vi "dataAcq_get_spectrum.vi"(0 "reference":refnum<class "OSA.lvclass">, 5 "error in (no error)":errorcluster, 9 "x data create":bool) -> (14 "duplicate reference":refnum<class "OSA.lvclass">, 19 "error out":errorcluster)   [LabVIEW 2010, in "OSA.lvclass"]
doc: "Reads data from spectrometer and updates labview buffer spectrum Y array, X is either equidistant, (x min and max), or contains a full X-array. See buffer_get.vi for labview buffer data access.\n\nX: periods/cm\nY: mW absolute pwr, (pwr/resolution)"
uses:
  OSA.lvclass
  typeDef/xVal_option.ctl
  OSA20X_misc.lvlib
  FTSLib.dll
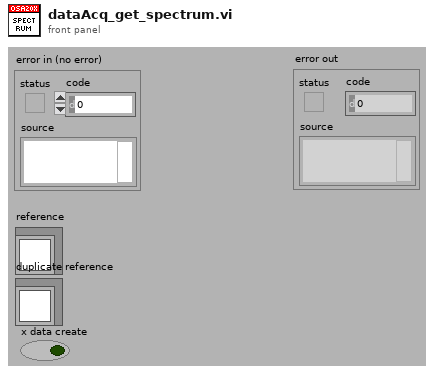
[diagram p1: front panel]
types:
  T1 = enum16{"get", "init", "set interferogram", "set spectrum", "cleanUp"}
  T2 = typedef "OSA.lvclass/ObjectAttributes.ctl" = cluster{"Stop":bool, "dataType":T3, "spectrometerIdx":u16, "buffer size interferogram":i32, "interferogram":cluster{"new":bool, "plot_x_ min":sgl, "plot_x_max":sgl, "plot_y_min":sgl, "plot_y_max":sgl, "Graph Intrfrgrm":T4, "timeStamp":u32, "signal (%)":dbl, "traces":cluster{"idx":u32, "broadBand":bool, "monoChromatic":bool, "peakToPeakSignal":dbl, "peakToPeakPos":dbl}[], "traces idx last":i32}, "spectrum":cluster{"new":bool, "plot_x_min":sgl, "plot_x_max":sgl, "plot_unit_x":T5, "plot_unit_y":T6, "plot_y_min":sgl, "plot_y_max":sgl, "Graph Spectrum":T4, "timeStamp":u32, "X_VAL_OPTIONS":enum16{"MIN_MAX", "ARRAY"}, "traces":cluster{"idx":u32}[], "traces idx last":i32}, "Thorlabs_OSA_64.lvclass:queue_action.ctlqueue ref":refnum<queue>, "action":T7, "plot zoom step":dbl, "buffer semaphore":T8, "acq stopped":bool, "dataType active":T3, "temperature (degr C)":sgl, "pressure (hPa)":sgl, "rel humidity (%)":sgl, "settings":cluster{"resolution":T9, "sensitivity":T10, "Average":bool, "average nr":u32, "apodisation":T11, "acq delay (ms)":u32, "airMesure":T12, "wmtr on":bool, "intfgrm_smooth_width":u16, "intfgrm_smooth_nrOfPasses":u16, "intfgrm_smooth":T13, "phaseCorrection":T14, "zeroFill":u8, "spectr_smooth":T13, "spectr_smooth_width":u16, "spectr_smooth_nrOfPasses":u16, "resolution (/cm)":sgl, "REF wavelength, (nm)":dbl, "gain_idx":u16, "gainAuto":bool, "gain_relative":dbl, "PD sensitivity mode":T15, "PD senseMode implemented":bool, "SensorTemperature implemented":bool, "SensorPressure implemented":bool, "SensorHumidity implemented":bool}, "peaks position":sgl[], "peaks width":sgl[], "peaks height":sgl[], "peaks max nr":u32, "peaks latest nr":i32, "peaks new":bool, "power":dbl, "power new":bool, "path":string, "wavelength (WNr)":dbl, "wavelength new":bool, "buffer size spectrum":i32, "status":string, "VI reference":refnum<vi>, "funcPointer":u64, "libraryPointer":u64, "singleAcquisition":bool, "coherenceLength (cm)":dbl, "coherenceLength new":bool, "spectrometer model":string, "spectrometer serial nr":string, "peaks thld left":sgl[], "peaks thld right":sgl[], "coherenceLength error (cm)":dbl, "ADC bits":u16, "peaks position centroid":sgl[], "peaks height centroid":sgl[], "OSA series":T16, "channel index":u16, "channel index stiched":u16, "spectrum channel type":T17}
  T3 = typedef "OSA.lvclass/acq_dataType.ctl" = enum16{"none", "interferogram", "spectrum"}
  T4 = typedef "OSA.lvclass/graph_intensity.ctl" = refnum<vi>
  T5 = typedef "OSA.lvclass/spectrum_x_unit.ctl" = enum16{"wavenr/cm", "THz", "eV", "nm_air", "nm_vac"}
  T6 = typedef "OSA.lvclass/y_unit.ctl" = enum16{"ADC counts", "dBm pwr absolute", "dBm pwr density", "mW pwr absolute", "mW pwr density"}
  T7 = typedef "OSA.lvclass/queue_action.ctl" = enum16{"none", "stop", "GUI_plotInterferogram", "GUI_plotSpectrum", "GUI_plotInterferogramRescale", "GUI_plotSpectrumRescale", "GUI_plotInterferogramReset", "GUI_plotSpectrumReset", "GUI_plotInterferogramAutoScaleY", "GUI_plotSpectrumAutoScaleY", "GUI_plotInterferogramZoomOut", "GUI_plotSpectrumZoomOut", "GUI_plotInterferogramPane", "GUI_plotSpectrumPane", "GUI_plotInterferogramZoomMouse", "GUI_plotSpectrumZoomMouse", "ENVIRONMENT temperature", "ENVIRONMENT pressure", "MODE_resolution set", "MODE_resolution get", "MODE_sensitivity set", "MODE_sensitivity get", "MODE_PDTemperature set", "MODE_PDTemperature get", "REBOOT/RESET firmware", "ACQASYNC_acquireSingleSpectrum", "ACQASYNC_continuous start", "ACQASYNC_continuous stop\n", "ACQASYNC_get last interferogram", "ACQASYNC_get last spectrum", "ACQASYNC_get last waveNr", "ACQOPT_interferogram smoothing set", "ACQOPT_interferogram smoothing get", "ACQOPT_spectrum smoothing set", "ACQOPT_spectrum smoothing get", "ACQOPT_apodisation type set", "ACQOPT_apodisation type get", "ACQOPT_phase correction type set", "ACQOPT_phase correction type get", "ACQOPT_acqIntervall_set", "ACQOPT_acqIntervall_get", "ACQOPT_average spectrum set", "ACQOPT_average spectrum get", "ACQOPT_rolling average set", "ACQOPT_rolling average get", "ACQOPT_zero fill factor set", "ACQOPT_zero fill factor get", "ACQOPT_cycle counting set", "ACQOPT_cycle counting get", "ACQOPT_air measure option set", "ACQOPT_air measure option get", "ACQOPT_gainLevel auto get", "ACQOPT_gainLevel auto set", "ACQOPT_gainLevel get", "ACQOPT_gainLevel set", "ACQOPT_getAll", "INSTRUMENT_PROPERTY_range_WaveNr_min", "INSTRUMENT_PROPERTY_range_WaveNr_max", "INSTRUMENT_PROPERTY_reference_wavelength_cm^-1", "INSTRUMENT_PROPERTY_samplesPerRefPeriod", "INSTRUMENT_PROPERTY_resolution_waveNrPercm", "INSTRUMENT_PROPERTY_availableGainLevels", "INSTRUMENT_PROPERTY_status", "CONVERT", "ANALYSE_POWER", "ANALYSE_PEAKS", "ANALYSE_WAVELENGTH", "ANALYSE_SPECTRUM", "ANALYSE_INTERFEROGRAM", "ANALYSE_COHERENCE_LENGTH", "MATH", "MATH_power", "MATH_peaks", "FILE", "miscellaneous"}
  T8 = typedef "Semaphore RefNum" = refnum<k1>
  T9 = typedef "OSA.lvclass/resolution.ctl" = enum16{"low", "high"}
  T10 = typedef "OSA.lvclass/sensitivityMode.ctl" = enum16{"low", "low medium", "high medium", "high"}
  T11 = typedef "OSA.lvclass/apodisation.ctl" = enum16{"NONE", "NORTON_BEER_WEAK", "NORTON_BEER_MEDIUM", "NORTON_BEER_STRONG", "TRIANGULAR", "COSINE", "HANN", "HAMMING", "BLACKMANHARRIS3", "BLACKMANHARRIS4", "GAUSSIAN"}
  T12 = typedef "OSA.lvclass/airMeasure.ctl" = enum16{"TEMPERATURE", "PRESSURE"}
  T13 = typedef "OSA.lvclass/smoothing.ctl" = enum16{"NONE", "BINOMIAL", "SAVITSKY_GOLAY", "FOURIER", "MOVING_AVERAGE", "GAUSSIAN"}
  T14 = typedef "OSA.lvclass/phaseCorrection.ctl" = enum16{"NONE", "MERTZ", "FORMAN", "MERTZ_FILE", "FORMAN_FILE", "FUTURE COMP."}
  T15 = typedef "OSA.lvclass/PDTemperatureMode.ctl" = enum16{"cool: better sensitivity/noise floor", "warm: extended wl range"}
  T16 = typedef "OSA.lvclass/OSA_series.ctl" = enum16{"OSA200", "OSA300", "UNKNOWN"}
  T17 = typedef "OSA.lvclass/channelType_spectrum.ctl" = enum16{"SINGLE CHANNEL", "STICHED"}
  T18 = typedef "OSA.lvclass/xVal_option.ctl" = enum16{"MIN_MAX", "ARRAY"}
  T19 = cluster{"length":u32, "X min":sgl, "X max":sgl, "X_VAL_OPTIONS":T18}
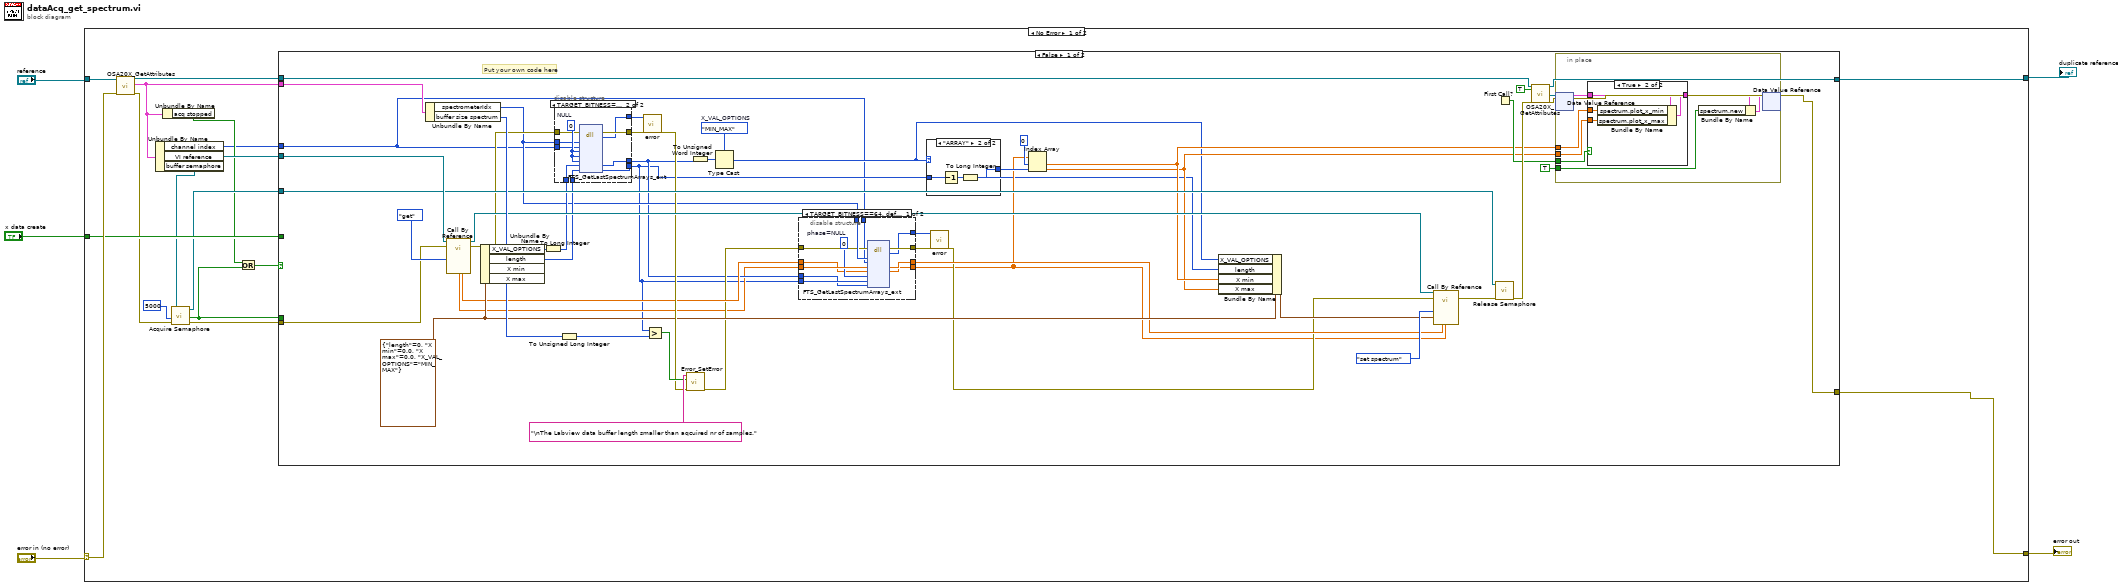
[diagram p0: block diagram]
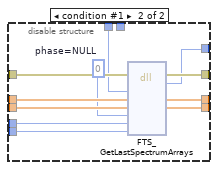
[diagram p2: hidden frame]
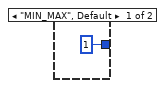
[diagram p3: hidden frame]
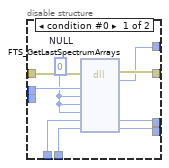
[diagram p4: hidden frame]
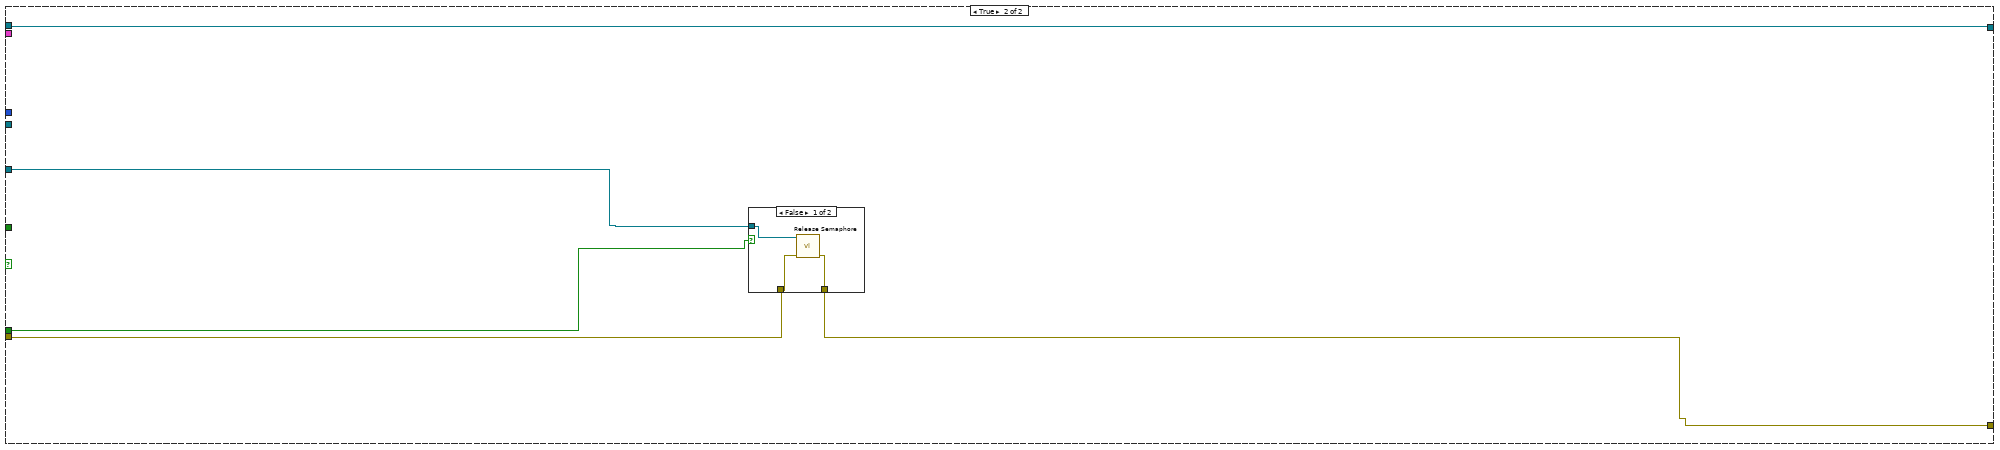
[diagram p6: hidden frame]
diagram:
  n1 = case shown="No Error" "error in (no error)" {
    selector: "error in (no error)" -> [w21 w139]
    tunnel: [w18 w139] -> w4
    tunnel: "reference" -> [w22 w138]
    tunnel: [w19 w138] -> w2
    tunnel: "x data create" -> [w20 _]
    frame No Error {
      n2 = call "OSA20X_GetAttributes.vi"("reference in"=w22, "error in (no error)"=w21) -> ("reference out"=w12:refnum<class "OSA.lvclass">, "Data"=w7:T2, "error out"=w16:errorcluster)  [unwired: 14 in, 1 out]
      n3 = Unbundle By Name(w7) -> ("channel index"=w6:u16, "VI reference"=w13:refnum<vi>, "buffer semaphore"=w14:T8)
      n4 = Unbundle By Name(w7) -> ("acq stopped"=w10:bool)
      n5 = call <vilib>:"Acquire Semaphore.vi"("error in (no error)"=w16, "ms timeout (-1)"=5000, "semaphore"=w14) -> ("error out"=w15:errorcluster, "timed out"=w8:bool, "semaphore out"=w11:T8)  [unwired: 2 in]
      n6 = Or(x=w10, y=w8) -> (x .or. y?=w9:bool)
      n7 = case shown="False" w9 {
        tunnel: w7 -> [w70 _]
        tunnel: w12 -> [w54 w133]
        tunnel: w20 -> [_ _]
        tunnel: [w66 w133] -> w19
        tunnel: [w65 w131] -> w18
        tunnel: w15 -> [w62 w132]
        tunnel: w13 -> [w61 _]
        tunnel: w11 -> [w58 w130]
        tunnel: w8 -> [_ w129]
        tunnel: w6 -> [w23 _]
        frame False {
          w40 = xVal_option."MIN_MAX"  # X_VAL_OPTIONS
          w44 = T19 {"length"=0, "X min"=0.0, "X max"=0.0, "X_VAL_OPTIONS"=enum."MIN_MAX"} ("spectrum property")
          # "Put your own code here"
          n8 = Unbundle By Name(w70) -> ("spectrometerIdx"=w38:u16, "buffer size spectrum"=w67:i32)
          n9 = call-by-ref "?"(reference=w61, error in=w62, "action"=T1."get") -> (reference out=w55:refnum<vi>, error out=w49:errorcluster, "spectrum X"=w34:sgl[], "spectrum Y"=w39:sgl[])  [unwired: 14 in, 3 out]
          n10 = Unbundle By Name(w44) -> ("X_VAL_OPTIONS"=w43:T18, "length"=w48:u32)  [unwired: 2 out]
          n11 = To Long Integer(number=w43) -> (32bit integer=w42:i32)
          n12 = disable-structure shown="TARGET_BITNESS==64, default" {
            disable-tunnel: w49 -> [w104 w115]
            disable-tunnel: w38 -> [w99 w113]
            disable-tunnel: [w101 w110] -> w24
            disable-tunnel: [w103 w114] -> w47
            disable-tunnel: w48 -> [w105 w112]
            disable-tunnel: [w102 w111] -> w45
            disable-tunnel: w42 -> [w106 w109]
            disable-tunnel: [w100 w108] -> w36
            disable-tunnel: w23 -> [_ w107]
            frame condition #0 {
              w98 = u32 0  # NULL
              n13 = dll-call lib="FTSLib.dll" fn="FTS_GetLastSpectrumArrays"(error in=w104, "spectrIdx"=w99, "spec"=w98, "x_data"=w98, "phase"=w98, "x_valueFormat"=w106, "length"=w105) -> (error out=w103:errorcluster, "return type"=w102:i32, "x_valueFormat"=w100:i32, "length"=w101:u32)  [unwired: 6 in, 1 out]
            }
            frame condition #1 (active) {
              w116 = u64 0  # NULL
              n14 = dll-call lib="FTSLib.dll" fn="FTS_GetLastSpectrumArrays_ext"(error in=w115, "spectrIdx"=w113, "channel"=w107, "spec"=w116, "x_data"=w116, "phase"=w116, "x_valueFormat"=w109, "length"=w112) -> (error out=w114:errorcluster, "return type"=w111:i32, "x_valueFormat"=w108:i32, "length"=w110:u32)  [unwired: 7 in, 1 out]
            }
          }
          n15 = To Unsigned Long Integer(number=w67) -> (unsigned 32bit integer=w64:u32)
          n16 = call "error.vi"("result code"=w45, "error in (no error)"=w47) -> ("error out"=w46:errorcluster)  [unwired: 15 in, 2 out]
          n17 = Greater?(x=w24, y=w64) -> (0:w68:bool)
          n18 = call "Error_SetError.vi"("error in"=w46, "status (true)"=w68, "source(\"\")"="\nThe Labview data buffer length smaller than aqcuired nr of samples." ("source(\"\")")) -> ("error out"=w37:errorcluster)  [unwired: 4 in]
          n19 = To Unsigned Word Integer(number=w36) -> (unsigned 16bit integer=w41:u16)
          n20 = Type Cast(type=w40, x=w41) -> (*(type *) &x=w25:T18)
          n21 = disable-structure shown="TARGET_BITNESS==64, default" {
            disable-tunnel: w39 -> [w82 w90]
            disable-tunnel: w38 -> [w81 w84]
            disable-tunnel: w37 -> [w80 w85]
            disable-tunnel: w36 -> [w78 w93]
            disable-tunnel: [w77 w89] -> w35
            disable-tunnel: w34 -> [w76 w91]
            disable-tunnel: [w75 w87] -> w33
            disable-tunnel: [w74 w86] -> w32
            disable-tunnel: w24 -> [w73 w92]
            disable-tunnel: [w72 w88] -> w26
            disable-tunnel: w23 -> [w71 _]
            frame condition #0 (active) {
              w79 = u64 0  # phase=NULL
              n22 = dll-call lib="FTSLib.dll" fn="FTS_GetLastSpectrumArrays_ext"(error in=w80, "spectrIdx"=w81, "channel"=w71, "spec"=w82, "x_data"=w76, "phase"=w79, "x_valueFormat"=w78, "length"=w73) -> (error out=w75:errorcluster, "return type"=w74:i32, "spec"=w77:sgl[], "x_data"=w72:sgl[])  [unwired: 7 in, 1 out]
            }
            frame condition #1 {
              w83 = u32 0  # phase=NULL
              n23 = dll-call lib="FTSLib.dll" fn="FTS_GetLastSpectrumArrays"(error in=w85, "spectrIdx"=w84, "spec"=w90, "x_data"=w91, "phase"=w83, "x_valueFormat"=w93, "length"=w92) -> (error out=w87:errorcluster, "return type"=w86:i32, "spec"=w89:sgl[], "x_data"=w88:sgl[])  [unwired: 6 in, 1 out]
            }
          }
          n24 = case shown="\"ARRAY\"" w25 {
            tunnel: w24 -> [_ w96]
            tunnel: [1 w95] -> w29
            frame "MIN_MAX", Default {
            }
            frame "ARRAY" {
              n25 = Decrement(x=w96) -> (x-1=w97:u32)
              n26 = To Long Integer(number=w97) -> (32bit integer=w95:i32)
            }
          }
          n27 = call "error.vi"("result code"=w32, "error in (no error)"=w33) -> ("error out"=w31:errorcluster)  [unwired: 15 in, 2 out]
          n28 = Index Array(array=w26, index #1=0 ("index"), index #2=w29) -> (element #1=w28:sgl, element #2=w27:sgl)
          n29 = Bundle By Name(cluster=w44, "X_VAL_OPTIONS"=w25, "length"=w24, "X min"=w28, "X max"=w27) -> (w56:T19)
          n30 = call-by-ref "?"(reference=w55, error in=w31, "action"=T1."set spectrum", "spectrum prop set"=w56, "spectrum set Y"=w35, "spectrum set X"=w26) -> (error out=w60:errorcluster)  [unwired: 11 in, 6 out]
          n31 = call <vilib>:"Release Semaphore.vi"("error in (no error)"=w60, "semaphore"=w58) -> ("error out"=w57:errorcluster)  [unwired: 4 in, 1 out]
          n32 = First Call?() -> (First Call?: T/F=w51:bool)
          n33 = call "OSA20X_GetAttributes.vi"("reference in"=w54, "OnlyGetDvrReference(False)"=TRUE, "error in (no error)"=w57) -> ("reference out"=w66:refnum<class "OSA.lvclass">, "DataRef"=w52:refnum<data-value>, "error out"=w65:errorcluster)  [unwired: 13 in, 1 out]
          n34 = in-place {
            in-place-border: w51 -> [w123]
            in-place-border: w28 -> [w121]
            in-place-border: w27 -> [w120]
            in-place-border: TRUE ("dataNewIntrfrgrm") -> [w118]
            n35 = in-place-dvr #1(w52) -> (w122:T2)  [unwired: 1 out]
            n36 = case shown="True" w123 {
              tunnel: w122 -> [w124 w128]
              tunnel: [w124 w127] -> w119
              tunnel: w121 -> [_ w126]
              tunnel: w120 -> [_ w125]
              frame False {
              }
              frame True {
                n37 = Bundle By Name(cluster=w128, "spectrum.plot_x_min"=w126, "spectrum.plot_x_max"=w125) -> (w127:T2)
              }
            }
            n38 = Bundle By Name(cluster=w119, "spectrum.new"=w118) -> (w117:T2)
            n39 = in-place-dvr #1(w117) -> ()  [unwired: 2 out]
          }
        }
        frame True {
          n40 = case shown="False" w129 {
            tunnel: w132 -> [w136 w137]
            tunnel: [w135 w137] -> w131
            tunnel: w130 -> [w134 _]
            frame False {
              n41 = call <vilib>:"Release Semaphore.vi"("error in (no error)"=w136, "semaphore"=w134) -> ("error out"=w135:errorcluster)  [unwired: 4 in, 1 out]
            }
            frame True {
            }
          }
        }
      }
    }
    frame Error {
      # "Error"
    }
  }
  "error out" <- w4
  "duplicate reference" <- w2
